vi "Add to Registry.vi"(8 "error in (no error)":errorcluster, 9 "iCVT_Item in":refnum<class "iCVT_Item.lvclass">, 10 "Tag Name":string, 11 "Current Value Table in":refnum<class "Current Value Table.lvclass">) -> (0 "error out":errorcluster, 2 "key already included?":bool, 3 "Current Value Table out":refnum<class "Current Value Table.lvclass">)   [LabVIEW 2024, in "Current Value Table.lvlib" / "Current Value Table.lvclass"]
uses:
  Current Value Table.lvclass
  iCVT_Item/iCVT_Item.lvclass
  Current Value Table.lvclass/Current Value Table.ctl
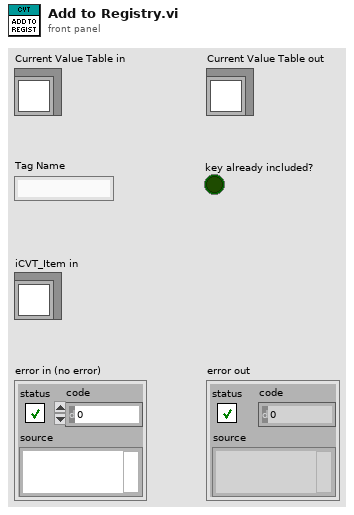
[diagram p1: front panel]
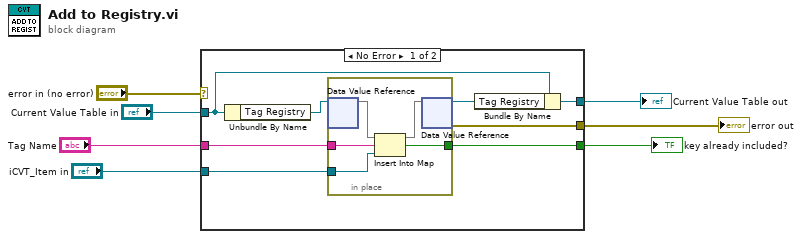
[diagram p0: block diagram]
diagram:
  n1 = case shown="No Error" "error in (no error)" {
    selector: "error in (no error)" -> [_ w22]
    tunnel: [w8 w22] -> w6
    tunnel: [w10 w21] -> w4
    tunnel: "Current Value Table in" -> [w12 w21]
    tunnel: "Tag Name" -> [w14 _]
    tunnel: "iCVT_Item in" -> [w13 _]
    tunnel: [w9 _] -> w1
    frame No Error {
      n2 = Unbundle By Name(w12) -> ("Tag Registry"=w15:refnum<data-value>)
      n3 = in-place {
        in-place-border: w14 -> [w19]
        in-place-border: w13 -> [w18]
        in-place-border: [w16] -> w9
        n4 = in-place-dvr #1(w15) -> (w20:map{string, refnum<class "iCVT_Item.lvclass">})  [unwired: 1 out]
        n5 = Insert Into Map(map in=w20, key=w19, value=w18) -> (map out=w17:map{string, refnum<class "iCVT_Item.lvclass">}, key already included?=w16:bool)  [unwired: 1 out]
        n6 = in-place-dvr #1(w17) -> (w11:refnum<data-value>, w8:errorcluster)
      }
      n7 = Bundle By Name(cluster=w12, "Tag Registry"=w11) -> (w10:refnum<class "Current Value Table.lvclass">)
    }
    frame Error {
    }
  }
  "error out" <- w6
  "Current Value Table out" <- w4
  "key already included?" <- w1
